vi "Sequence Specialdata inquiry.vi"(7 "Channel  (1: CH1)":u16(ring)=1 items=["CH1"=1, "CH2"=2, "CH3"=3, "CH4"=4], 8 "error in (no error)":errorcluster, 11 "VISA resource name":refnum<visa-resource-name>) -> (0 "error out":errorcluster, 1 "Rise Rate":dbl, 2 "Fall Rate":dbl, 3 "VISA resource name out":refnum<visa-resource-name>, 4 "Width(Pulse)":dbl, 6 "Symmetry(Ramp)":dbl)   [LabVIEW 2020, in "GPP.lvlib"]
uses:
  GPP.lvlib
  Function/VISA_COMMON.ctl
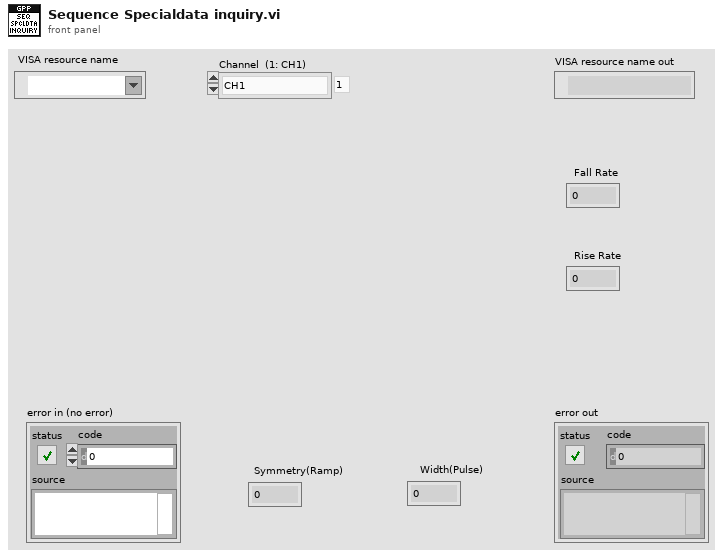
[diagram p1: front panel]
types:
  T1 = typedef "GPP.lvlib/VISA_COMMON.ctl" = enum16{"Initial", "Write CMD", "Read Result", "Read History", "Close"}
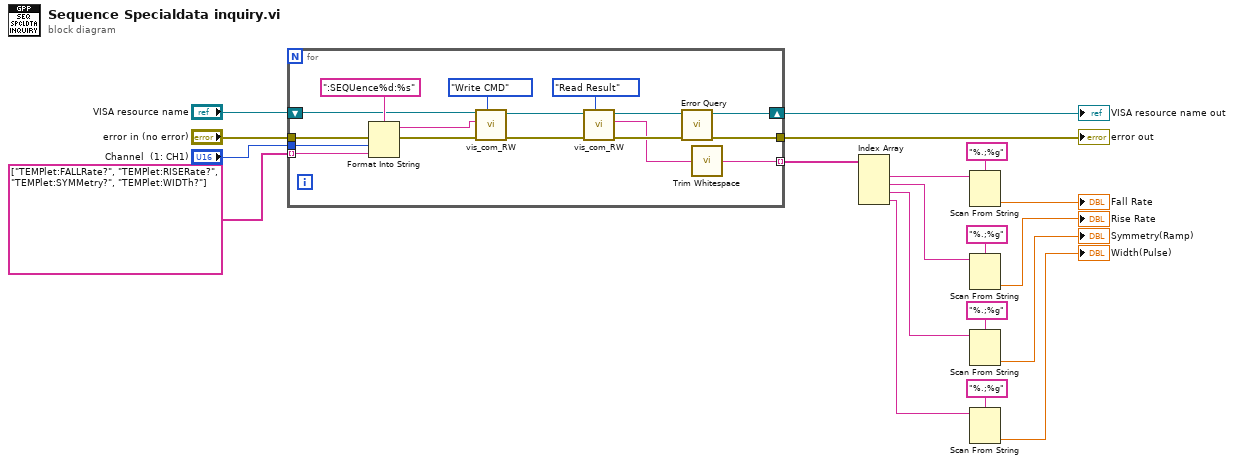
[diagram p0: block diagram]
diagram:
  n1 = for {
    tunnel: "error in (no error)" -> [w30]
    tunnel: "Channel  (1: CH1)" -> [w28]
    tunnel: string[] ["TEMPlet:FALLRate?", "TEMPlet:RISERate?", "TEMPlet:SYMMetry?", "TEMPlet:WIDTh?"] -> [w25] mode=indexing
    tunnel: [w26] -> w10
    tunnel: [w22] -> w16 mode=indexing
    shift-right: [w20] -> w9
    shift-left: "VISA resource name" -> [w24]
    n2 = Format Into String(format string=":SEQUence%d:%s", error in=w30, w28, w25) -> (resulting string=w23:string, error out=w29:errorcluster)  [unwired: 1 in]
    n3 = call "vis_com_RW.vi"("Funciton"=VISA_COMMON."Write CMD", "error in (no error)"=w29, "CMD String"=w23, "VISA resource in"=w24) -> ("error out"=w34:errorcluster, "VISA resource out"=w33:refnum<visa-resource-name>)  [unwired: 5 in, 1 out]
    n4 = call "vis_com_RW.vi"("Funciton"=VISA_COMMON."Read Result", "error in (no error)"=w34, "VISA resource in"=w33) -> ("error out"=w31:errorcluster, "Result"=w21:string, "VISA resource out"=w32:refnum<visa-resource-name>)  [unwired: 6 in]
    n5 = call "Error Query.vi"("error in (no error)"=w31, "VISA resource name"=w32) -> ("error out"=w26:errorcluster, "VISA resource name out"=w20:refnum<visa-resource-name>)  [unwired: 6 in, 2 out]
    n6 = call <vilib>:"Trim Whitespace.vi"("string"=w21) -> ("trimmed string"=w22:string)  [unwired: 1 in]
  }
  "error out" <- w10
  "VISA resource name out" <- w9
  n7 = Index Array(array=w16) -> (element #1=w7:string, element #2=w13:string, element #3=w12:string, element #4=w5:string)  [unwired: 4 in]
  n8 = Scan From String(format string="%.;%g", input string=w7) -> (output 1=→"Fall Rate":dbl)  [unwired: 3 in, 3 out]
  n9 = Scan From String(format string="%.;%g", input string=w13) -> (output 1=→"Rise Rate":dbl)  [unwired: 3 in, 3 out]
  n10 = Scan From String(format string="%.;%g", input string=w12) -> (output 1=→"Symmetry(Ramp)":dbl)  [unwired: 3 in, 3 out]
  n11 = Scan From String(format string="%.;%g", input string=w5) -> (output 1=→"Width(Pulse)":dbl)  [unwired: 3 in, 3 out]
